vi "Query Output.vi"(8 "error in":errorcluster, 11 "ProXR_IO in":refnum<class "ProXR.lvclass">) -> (0 "error out":errorcluster, 1 "Digital Out":bool[](array[boolean]), 2 "Query All Banks":u8[](array[numeric]), 3 "ProXR_IO out":refnum<class "ProXR.lvclass">)   [LabVIEW 2019, in "ProXR.lvlib" / "ProXR.lvclass"]
uses:
  Library/ProXR.lvclass
  C:/Users/Public/Documents/Development/builds/Instruments/DIG_IO.lvlibp/Library/DIG_IO.lvclass
  builds/Instruments/DIG_IO.lvlibp/Accessors/Read Control.vi
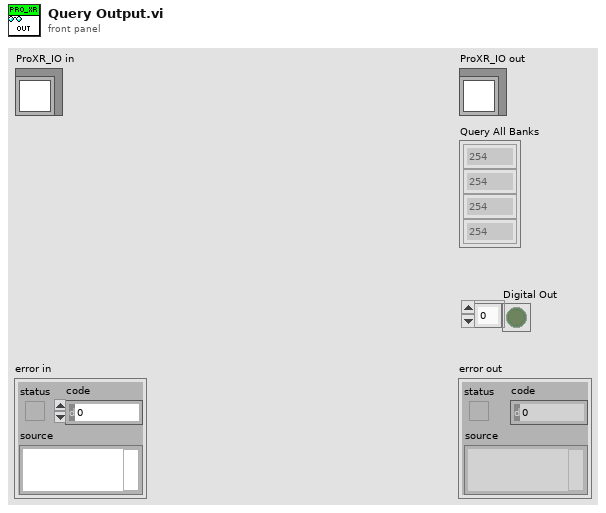
[diagram p1: front panel]
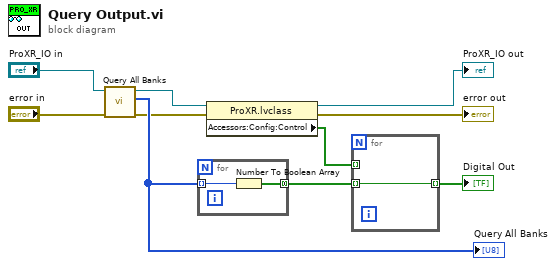
[diagram p0: block diagram]
diagram:
  n1 = call "Query All Banks.vi"("error in"="error in", "ProXR_IO in"="ProXR_IO in") -> ("error out"=w5:errorcluster, "Query All Banks"=w10:u8[], "ProXR_IO out"=w7:refnum<class "ProXR.lvclass">)  [unwired: 7 in]
  "Query All Banks" <- w10
  n2 = for {
    tunnel: w10 -> [w12] mode=indexing
    tunnel: [w11] -> w2 mode=concatenating
    n3 = Number To Boolean Array(number=w12) -> (Boolean array=w11:bool[])
  }
  n4 = property class="ProXR.lvclass"(reference=w7, error in=w5) -> (reference out=→"ProXR_IO out":refnum<class "ProXR.lvclass">, error out=→"error out":errorcluster, "Accessors:Config:Control"=w1:bool[])
  n5 = for {
    tunnel: [w13] -> w3 mode=indexing
    tunnel: w2 -> [w13] mode=indexing
    tunnel: w1 -> [_] mode=indexing
  }
  "Digital Out" <- w3
